vi "Setup UI.vi"(8 "error in (no error)":errorcluster, 10 "Set UI to input? (F)":bool, 11 "Dummy Scan in":refnum<class "Dummy Scan.lvclass">) -> (0 "error out":errorcluster, 3 "Dummy Scan out":refnum<class "Dummy Scan.lvclass">)   [LabVIEW 2017, in "Dummy Scan.lvclass"]
doc: "Scanner::Setup is a constructor that has no parameters and faces the user. The Factory calls this VI to let the user configure this Scanner. It is dynamically dispatched in order to let the user choose the type as well as the options of the scanner."
uses:
  Dummy Scan.lvclass
  Scanner/Scanner.lvclass
panel:
  # "Dummy Scan Setup"
  # "This dummy scanner has no options."
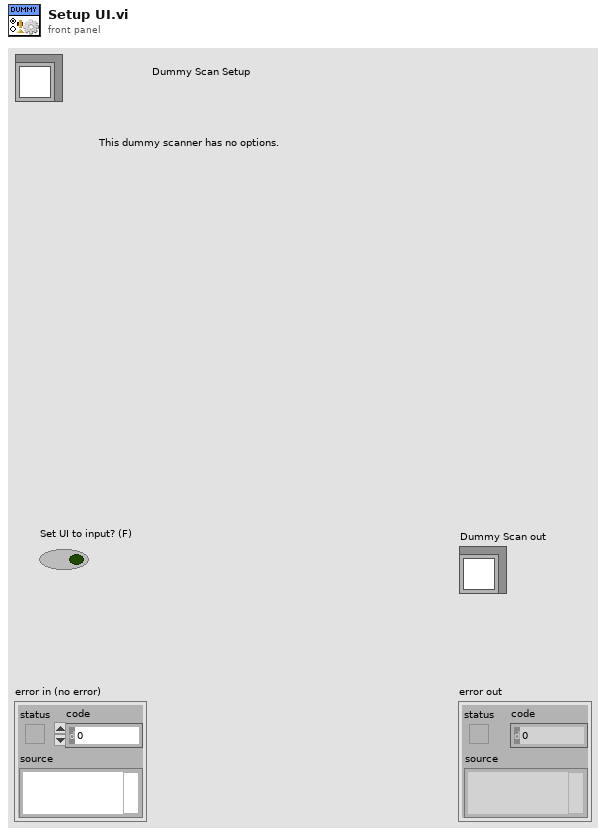
[diagram p1: front panel]
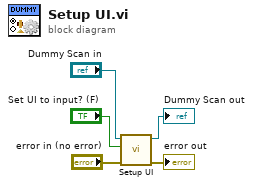
[diagram p0: block diagram]
diagram:
  n1 = call-parent "Setup UI.vi"("error in (no error)"="error in (no error)", "Set UI to input? (F)"="Set UI to input? (F)", "Scanner in"="Dummy Scan in") -> ("error out"=→"error out":errorcluster, "Scanner out"=→"Dummy Scan out":refnum<class "Dummy Scan.lvclass">)  [unwired: 7 in]
